vi "flushTel.vi"(8 "error in (no error)":errorcluster, 10 "queueName":enum16{"queueFromDds", "queueToDds"}(ring), 11 "tcpServerTel in":refnum<class "TcpServerTel.lvclass">) -> (0 "error out":errorcluster, 2 "telemetry flushed":string[](array[string]), 3 "tcpServerTel out":refnum<class "TcpServerTel.lvclass">)   [LabVIEW 2018, in "TcpServerTel.lvclass"]
doc: "Get all elements from either queueToDds or queueFromDds, using Flush Queue function. Use the queueName enum control to select the queue."
uses:
  TcpServerTel.lvclass
  home/pcortes/github/ts_labview_tcp_json/src/TcpServerBase/TcpServerBase.lvclass
  TcpServerTel.lvclass/TcpServerTel.ctl
  TcpServerBase/TcpServerBase.lvclass/TcpServerBase.ctl
  TcpServerBase/TcpServerBase.lvclass
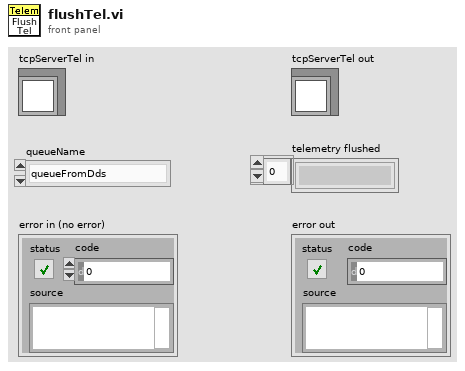
[diagram p1: front panel]
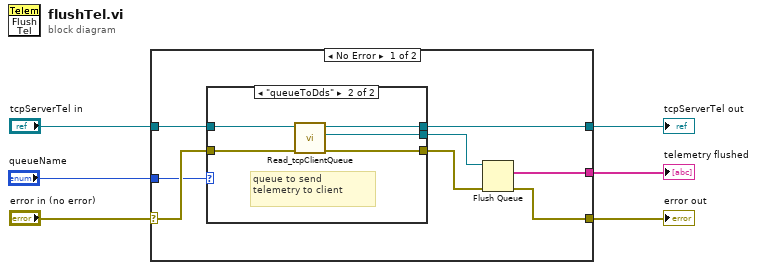
[diagram p0: block diagram]
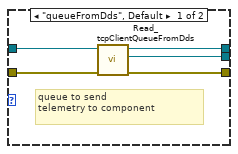
[diagram p2: hidden frame]
diagram:
  n1 = case shown="No Error" "error in (no error)" {
    selector: "error in (no error)" -> [w10 w26]
    tunnel: "tcpServerTel in" -> [w12 w25]
    tunnel: [w11 w25] -> w5
    tunnel: [w9 w26] -> w3
    tunnel: [w8 _] -> w2
    tunnel: "queueName" -> [w7 _]
    frame No Error {
      n2 = case shown="\"queueToDds\"" w7 {
        tunnel: [w19 w20] -> w14
        tunnel: [w18 w21] -> w13
        tunnel: w12 -> [w17 w24]
        tunnel: [w16 w23] -> w11
        tunnel: w10 -> [w15 w22]
        frame "queueFromDds", Default {
          # "queue to send\ntelemetry to component"
          n3 = call "Read_tcpClientQueueFromDds.vi"("error in (no error)"=w15, "TcpServerTel in"=w17) -> ("error out"=w18:errorcluster, "tcpClientQueueFromDds"=w19:refnum<queue>, "TcpServerTel out"=w16:refnum<class "TcpServerTel.lvclass">)  [unwired: 7 in]
        }
        frame "queueToDds" {
          # "queue to send\ntelemetry to client"
          n4 = call "Read_tcpClientQueue.vi"("error in (no error)"=w22, "TcpServerBase in"=w24) -> ("error out"=w21:errorcluster, "tcpClientQueue"=w20:refnum<queue>, "TcpServerBase out"=w23:refnum<class "TcpServerTel.lvclass">)  [unwired: 7 in]
        }
      }
      n5 = Flush Queue(queue=w14, error in (no error)=w13) -> (remaining elements=w8:string[], error out=w9:errorcluster)  [unwired: 1 out]
    }
    frame Error {
    }
  }
  "error out" <- w3
  "tcpServerTel out" <- w5
  "telemetry flushed" <- w2
